vi "STP_22.1 - three_multiAO+dynamics.vi"() -> ()   [LabVIEW 2018]
uses:
  <vilib>/Math Plots/2D Math Plots/2D Compass/2D Compass XCtrl/2D Compass.xctl
  <vilib>/Utility/error.llb/DialogType.ctl
  <vilib>/Platform/TimedLoop/XDataNode/nitl_modes.ctl
  <vilib>/Platform/TimedLoop/XDataNode/timing_clust.ctl
  <vilib>/Platform/TimedLoop/XDataNode/wakeup.ctl
  <vilib>/DAQmx/write.llb/DAQmx Write (Analog 1D Wfm NChan NSamp).vi
  <vilib>/DAQmx/write.llb/DAQmx Write (Analog 2D DBL NChan NSamp).vi
  <vilib>/DAQmx/create/timing.llb/DAQmx Create Timing Source (Frequency).vi
  <vilib>/Instr/_visa.llb/VISA Configure Serial Port (Instr).vi
  <vilib>/Math Plots/2D Math Plots/2D Compass/2D Compass Datatype/Public/Plot Helper (Vector).vi
  <vilib>/DAQmx/create/channels.llb/DAQmx Create Channel (AO-Voltage-Basic).vi
  <vilib>/DAQmx/configure/timing.llb/DAQmx Timing (Sample Clock).vi
  <vilib>/DAQmx/miscellaneous.llb/DAQmx Fill In Error Info.vi
  <vilib>/measure/matone.llb/Extract Single Tone Information 1 Chan.vi
  <vilib>/Platform/TimedLoop/XDataNode/XDataNode.xnode
  <vilib>/measure/NI_MABase.lvlib
  <resource>/objmgr/daqmx.rc
  <vilib>/Platform/TimedLoop/XDataNode/XDNodeRunTimeDep.lvlib
  <vilib>/measure/NI_MAPro.lvlib
  <vilib>/Math Plots/2D Math Plots/2D Compass/2D Compass Datatype/2D Compass Datatype.lvclass
  <vilib>/Analysis/NI_AALBase.lvlib
  <vilib>/Analysis/NI_AALPro.lvlib
panel:
  out "rocof0":dbl[](array[numeric])
  out "rocof1":dbl[](array[numeric])
  out "ROCOF measured":dbl[](array[numeric])
  out "ROCOF reference":dbl[](array[numeric])
  out "Media":dbl
  in  "stop":bool
  out "Frequency reference":dbl[](array[numeric])
  out "Frequency measured":dbl[](array[numeric])
  out "Angle reference":dbl[](array[numeric])
  out "Angle measured":dbl[](array[numeric])
  out "Voltage reference":dbl[](array[numeric])
  out "Voltage measured":dbl[](array[numeric])
  out "freq1":dbl[](array[numeric])
  out "freq0":dbl[](array[numeric])
  out "magnitude1":dbl[](array[numeric])
  out "magnitude0":dbl[](array[numeric])
  in  "last amp":dbl
  out "phases0":dbl[](array[numeric])
  out "phases1":dbl[](array[numeric])
  out "initialized array":dbl[](array[numeric])
  out "Sine phase":dbl
  in  "Tab Control":T1(tab)
  out "Interf.\nAmplitude (%)":dbl
  out "Interf.\nFrequency (Hz)":dbl
  out "Amplitude (%)":dbl
  out "Harmonic order":i32
  out "reset\nphase?":bool
  out "Samples":dbl
  out "Frequency (Hz)":dbl
  out "Phase (deg)":dbl format="%.4f"
  out "Amplitude (V)":dbl format="%.4g"
  in  "Tab Control 3":T2(tab)
  in  "Interference":bool
  in  "Interf. Frequency":dbl caption="Frequency"
  in  "Interf. Amplitude":dbl caption="Amplitude (%)"
  in  "Amplitude (%)":dbl=10.0
  in  "Order":i32=2
  in  "Harmonics":bool
  in  "phase 2":dbl
  in  "duty cycle (%)":dbl=1.0
  in  "Pulse frequency":dbl=25.0
  in  "Noise":bool
  in  "Amplitude (rms)":dbl=0.0035355 format="%0.6f"
  in  "reset signal":bool
  in  "Phase":dbl format="%#.4f"
  in  "Frequency":dbl=50.0 format="%#.4f"
  in  "Offset":dbl=1.5 format="%#.4f"
  in  "Amplitude":dbl=1.25 format="%#.4f"
  in  "Steps":dbl=50.0
  in  "Save without\nvariation":bool
  in  "Amp. (%) 4":dbl=10.0 caption="Amplitude (%)"
  in  "Frequency\ninterval 2":dbl=0.5 caption="Frequency\ninterval"
  in  "Final freq. 2":dbl=100.0 caption="Final freq."
  in  "Initial freq. 2":dbl=27.5 caption="Initial freq."
  in  "Interference\nauto variation":bool
  in  "Amp. (%) 3":dbl=10.0 caption="Amplitude (%)"
  in  "Order\ninterval":i32=1
  in  "Final order":i32=50
  in  "Initial order":i32=2
  in  "Harmonics\nauto variation":bool
  in  "Frequency\ninterval":dbl=0.1 format="%.4f"
  in  "Final freq.":dbl=55.0 format="%.4f"
  in  "Initial freq.":dbl=45.0 format="%.4f"
  in  "Freq. auto\nvariation":bool
  in  "Phase\ninterval":dbl=10.0 format="%.4f"
  in  "Final phase":dbl=180.0 format="%.4f"
  in  "Initial phase":dbl=-180.0 format="%.4f"
  in  "Phase auto\nvariation":bool
  in  "Amplitude\ninterval":dbl=0.05 format="%.4f"
  in  "Initial ampl.":dbl=0.125 format="%.4f"
  in  "Final ampl.":dbl=1.25 format="%.4f"
  in  "Ampl. auto\nvariation":bool
  in  "Boolean 2":bool
  in  "Dynamic tests?":bool
  in  "Final fmod":dbl=5.0
  in  "fmod interval":dbl=0.2
  in  "Initial fmod":dbl
  in  "Modulation\nauto variation":bool
  in  "Select test type":T3(ring)
  in  "Freq. Ramp":bool
  in  "ka":dbl=0.1
  in  "kx":dbl=0.1
  out "fmod (Hz)":dbl
  in  "fmod":dbl
  in  "Signal generation":bool=TRUE
  in  "File name":path=path "teste.txt"
  in  "Data save":bool
  in  "Boolean":bool
  in  "step time (s)":i32=2
  out "step?":bool
  out "Cycle visualization":dbl[](graph)
  in  "Boolean 3":bool
  out "Phasors visualization":refnum<class "2D Plot Datatype.lvclass">[](xcontrol) caption="2D Compass"
  in  "Directory":path=path "D:/Resultados"
  in  "Sampling rate":dbl=200000.0
  in  "Porta":refnum<visa-resource-name>="COM3"
  in  "baud rate (kB)":u32=115200
  in  "data bits (8)":u16=8
  in  "timeout (ms)":u32=5000
  in  "parity (0:none)":enum16{"None", "Odd", "Even", "Mark", "Space"}(ring)
  in  "flow control (0:none)":u16(ring) items=["None", "XON/XOFF", "RTS/CTS", "XON/XOFF & RTS/CTS", "DTR/DSR", "XON/XOFF & DTR/DSR"]
  in  "stop bits (10: 1 bit)":u16(ring)=10 items=["1.0"=10, "1.5"=15, "2.0"=20]
  in  "Serial communication":bool=TRUE
  out "read buffer":string
  out "floating point data":sgl[](array[numeric])
  in  "Interference 2":bool caption="Interference"
  in  "amplitude":dbl=1.0 caption="Amp. (%)" format="%#.4p"
  in  "Interf. Frequency 2":dbl=10.0 caption="Frequency (Hz)"
  in  "Harmonics 2":bool caption="Harmonics"
  in  "Amp. (%) 2":dbl=10.0 caption="Amp. (%)"
  in  "Order 2":i32=3 caption="Order"
  out "Frequency":dbl
  in  "Offset 2":dbl=1.5 caption="Offset"
  out "Phase (degrees) 2":dbl caption="Phase (°)" format="%.4f"
  in  "Amplitude 2":dbl=1.25 caption="Amplitude"
  in  "Frequency 2":dbl=50.0 caption="Frequency"
  in  "Phase 2":dbl caption="Phase"
  in  "reset signal 2":bool caption="reset\nsignal"
  in  "Frequency\noff-set":dbl
  in  "Magnitude\noff-set":dbl
  in  "Magnitude\ncoefficient":dbl=1.0
  in  "Angle\noff-set":dbl
  out "mean rocof":dbl caption="ROCOF (Hz/s)" format="%.8g"
  out "max rocof":dbl caption="ROCOF (Hz/s)" format="%.8g"
  out "mean freq":dbl caption="Frequency (Hz)" format="%.8g"
  out "mean tve":dbl caption="TVE (%)" format="%.8g"
  out "mean phase":dbl caption="Phase (º)" format="%.8g"
  out "mean dev":dbl caption="Magnitude (%)" format="%.8g"
  out "max magnitude":dbl caption="Magnitude (%)" format="%.8g"
  out "max tve":dbl caption="TVE (%)" format="%.8g"
  out "max freq":dbl caption="Frequency (Hz)" format="%.8g"
  out "max phase":dbl caption="Phase (º)" format="%.8g"
  in  "Tab Control 2":T4(tab)
  out "Magnitude measures (V)":dbl[][](graph)
  in  "?":bool
  in  "RMS?":bool=TRUE
  out "Phase measures (º)":dbl[][](graph)
  in  "?":bool
  in  "Fase ref":enum16{"R", "S", "T"}(ring)
  out "Frequency measures (Hz)":dbl[][](graph)
  in  "?":bool
  out "ROCOF (Hz/s)":dbl[][](graph)
  in  "?":bool
  in  "?":bool
  out "Phase measures (º) 2":dbl[](graph)
  out "Iteration Duration 2":i64
  out "Finished Late? [i-1]":bool
  out "Iteration Duration":i64
  out "Iteration Duration 3":i64
  # "Synchrophasors Test Platform"
  # "A real-time platform for PMU development."
  # "Actual generation"
  # "PPS parameters"
  # "Noise"
  # "Sinusoid parameters"
  # "1 Hz/s"
  # "IEEE 754 conversion"
  # "Max errors:"
  # "Mean errors:"
  # "Signal generation parameters:"
  # "On-line corrections (received data):"
  # "This is a project developed by Flavio Lori Grando, during Masters in Electrical Engineering Graduate Program (PPGEE) of Federal University of Technology - Paraná, Brazil.\n\nContact: flavio.grando.eng@gmail.com"
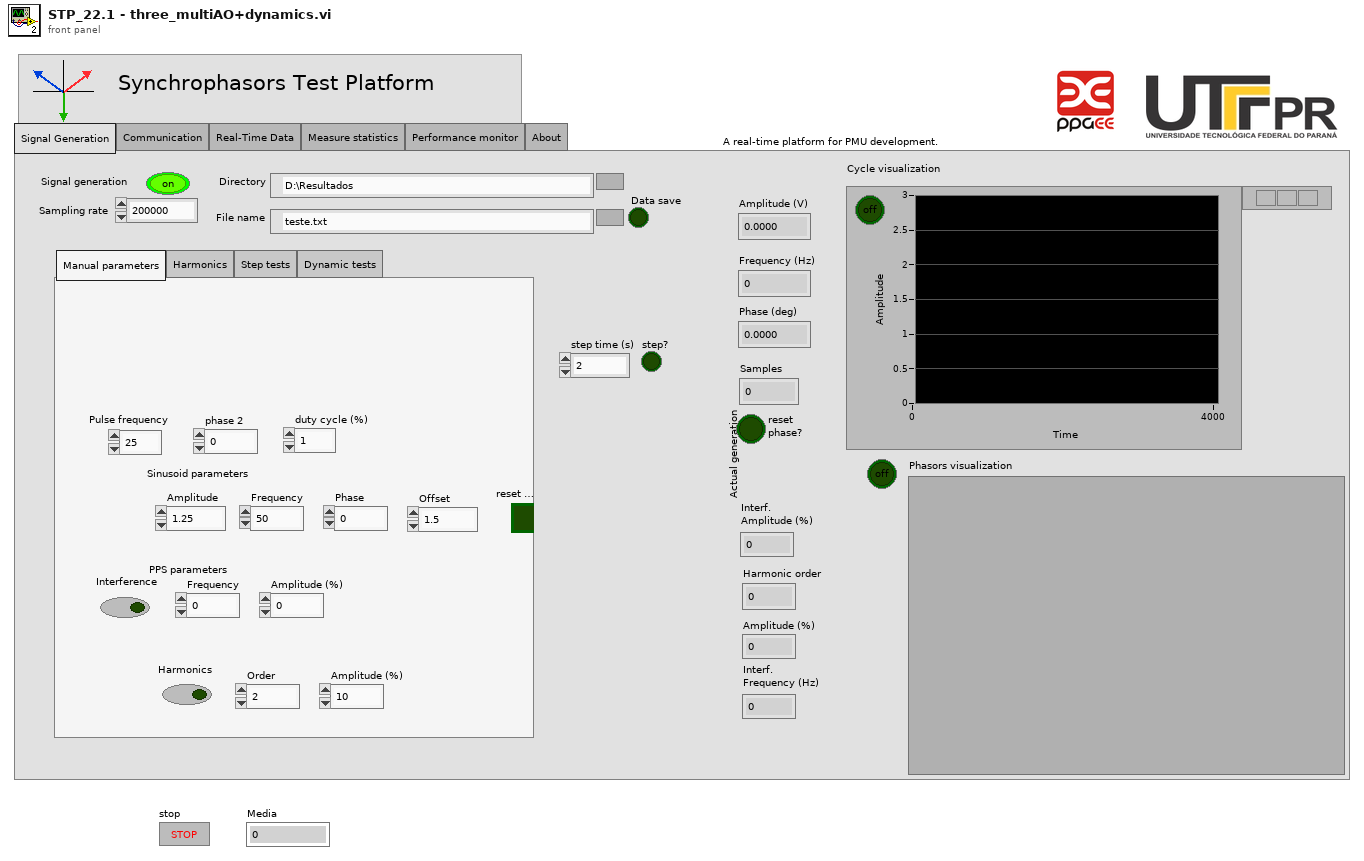
[diagram p1: front panel]
types:
  T1 = enum32{"Signal Generation", "Communication", "Real-Time Data", "Measure statistics", "Performance monitor", "About"}
  T2 = enum32{"Manual parameters", "Harmonics", "Step tests", "Dynamic tests"}
  T3 = enum16{"Amplitude modulation", "Phase modulation", "Frequency ramp"}
  T4 = enum32{"Magnitude", "Phase", "Frequency", "ROCOF", "Phase deviation"}
  T5 = enum16{"Sine Wave", "Triangle Wave", "Square Wave", "Sawtooth Wave"}
  T6 = typedef "XDNodeRunTimeDep.lvlib/nitl_modes.ctl" = enum32{"No Change", "Process missed periods, maintain original phase", "Discard missed periods, maintain original phase", "Process missed periods, ignore original phase", "Discard missed periods, ignore original phase"}
  T7 = cluster{"frequency":dbl, "amplitude":dbl, "phase":dbl}[]
  T8 = typedef "XDNodeRunTimeDep.lvlib/timing_clust.ctl" = cluster{"Expected End [f-1]":u64, "Actual End [f-1]":u64, "Finished Late? [f-1]":bool, "Expected End [i-1]":u64, "Actual End [i-1]":u64, "Finished Late? [i-1]":bool, "Expected Start [i]":u64, "Actual Start [i]":u64, "Expected Start [f]":u64, "Actual Start [f]":u64, "Source Name":string, "Structure Name":string, "Period":i64, "Deadline":i64, "Offset":i64, "Start":i64, "Priority":i32, "Timeout":i32, "Mode":T6, "Wakeup Reason":T9, "Error":errorcluster, "Source Type":string, "Secondary Source Type":string, "Global End Time":u64, "Global Start Time":u64, "Frame Duration":u64, "Iteration Duration":u64, "Assigned CPU":i32, "I/O Scan Engine Mode":u32}
  T9 = typedef "XDNodeRunTimeDep.lvlib/wakeup.ctl" = enum32{"Normal", "Aborted", "Asynchronous wakeup", "Timing source error", "Timed loop error", "Timeout"}
  T10 = typedef "DialogType.ctl" = u16
  T11 = cluster{"Sampling rate":dbl, "Sampling rate":dbl}
  T12 = enum16{"open", "replace", "create", "open or create", "replace or create", "replace or create with confirmation"}
  T13 = cluster{"max ref":dbl, "min ref":dbl, "mean ref":dbl, "max dev":dbl, "min dev":dbl, "mean dev":dbl, "max meas":dbl, "min meas":dbl, "mean meas":dbl}
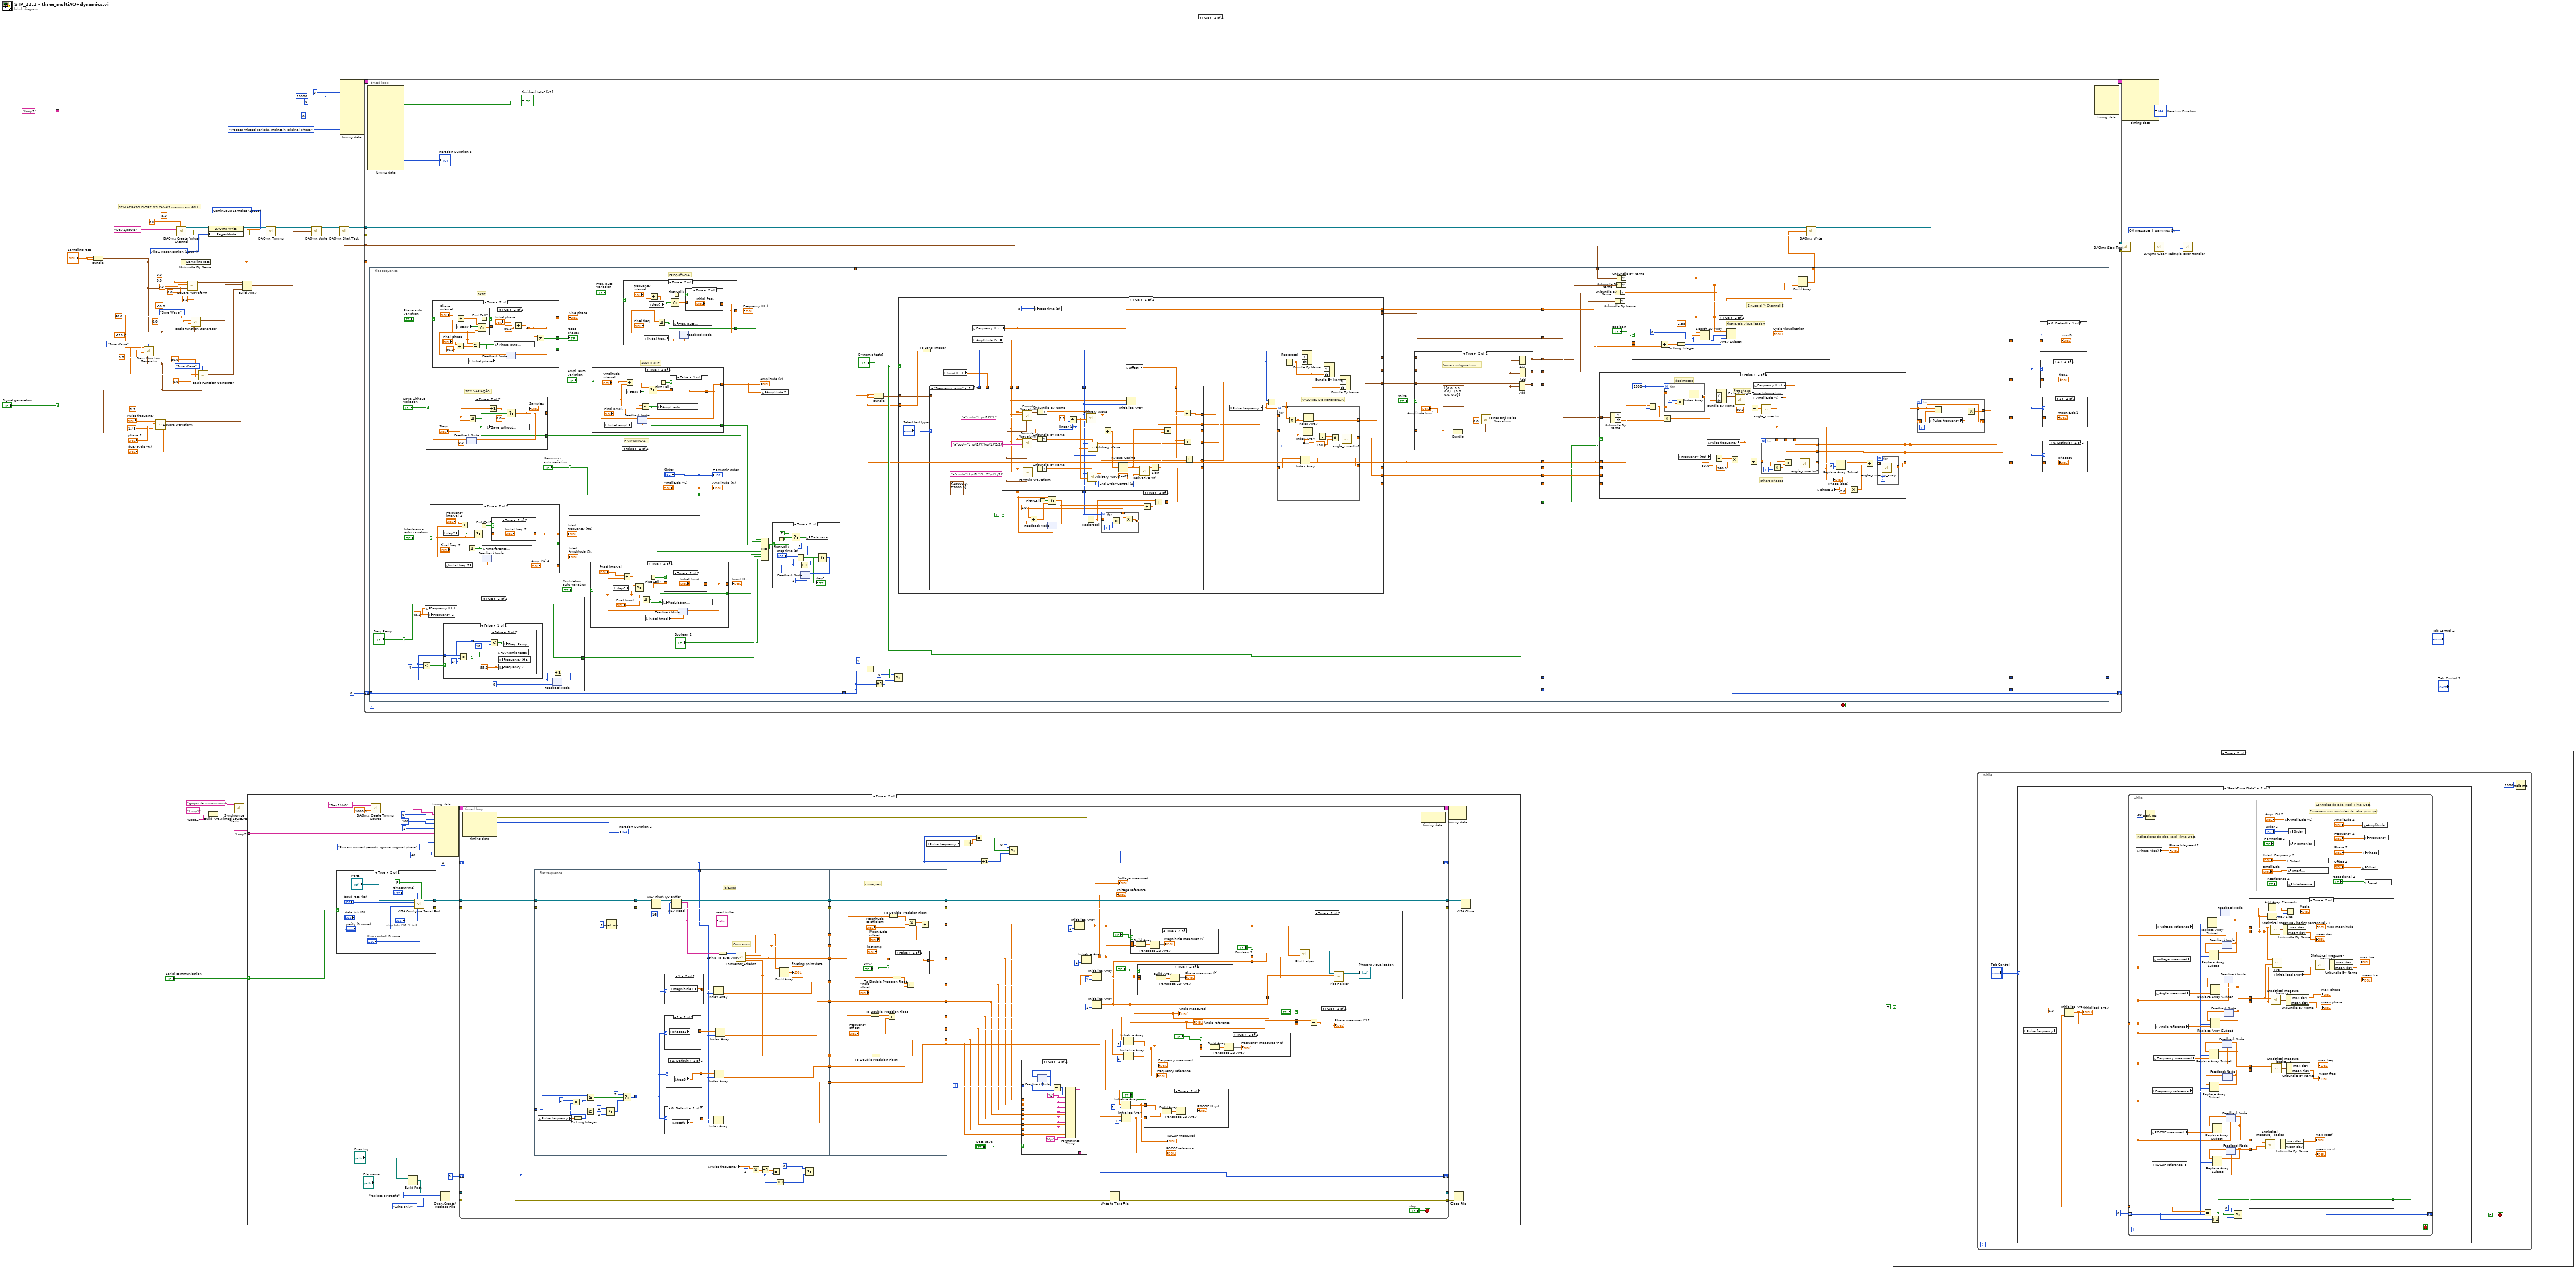
[diagram p0: block diagram]
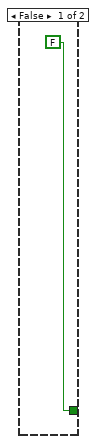
[diagram p4: hidden frame]
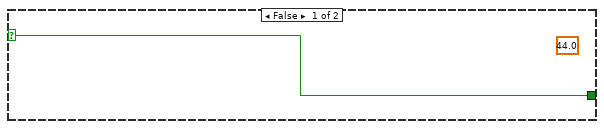
[diagram p7: hidden frame]
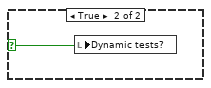
[diagram p8: hidden frame]
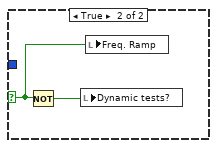
[diagram p9: hidden frame]
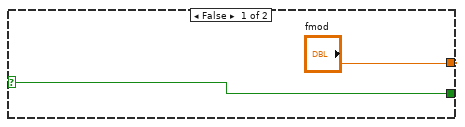
[diagram p10: hidden frame]
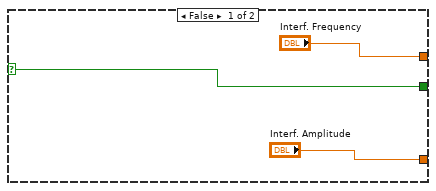
[diagram p12: hidden frame]
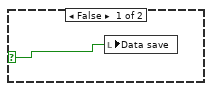
[diagram p14: hidden frame]
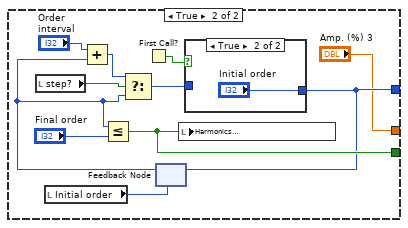
[diagram p15: hidden frame]
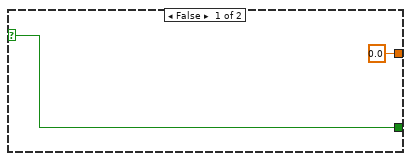
[diagram p17: hidden frame]
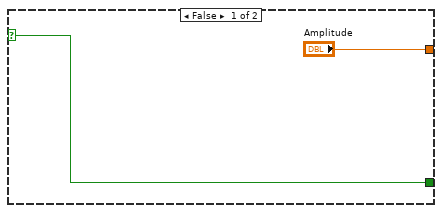
[diagram p18: hidden frame]
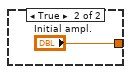
[diagram p19: hidden frame]
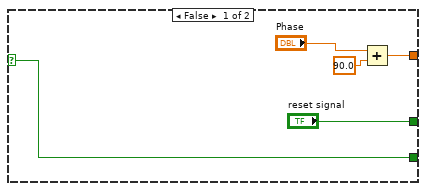
[diagram p20: hidden frame]
diagram:
  n1 = case shown="True" "Signal generation" {
    tunnel: "Loop1" -> [_ w33]
    frame False {
    }
    frame True {
      w20 = 60.0 ("frequency")
      w61 = 10097 items=["Allow Regeneration"=10097, "Do Not Allow Regeneration"=10158] ("RegenMode")
      w64 = 10123 items=["Finite Samples"=10178, "Continuous Samples"=10123] ("sample mode")
      w65 = T10 3 items=["no dialog", "OK message", "continue or stop message", "OK message + warnings", "continue/stop + warnings"] ("type of dialog (OK msg:1)")
      # "SEM ATRASO ENTRE OS CANAIS mesmo em 60Hz"
      n2 = Bundle("Sampling rate"="Sampling rate", "Sampling rate"="Sampling rate") -> (w11:T11)  [unwired: 1 in]
      n3 = call <vilib>:"Basic Function Generator.vi"("sampling info"=w11, "signal type"=T5."Sine Wave" ("signal type 4"), "phase"=-210.0 ("offset 4"), "amplitude"=0.0 ("amplitude 3"), "frequency"=w20) -> ("signal out"=w25:waveform(dbl))  [unwired: 4 in, 2 out]
      n4 = call <vilib>:"Square Waveform.vi"("duty cycle (%)"="duty cycle (%)", "offset"=1.5, "sampling info"=w11, "phase"="phase 2", "amplitude"=1.45, "frequency"="Pulse frequency") -> ("signal out"=w29:waveform(dbl))  [unwired: 4 in, 1 out]
      n5 = call-poly <vilib>:"DAQmx Create Virtual Channel.vi"("maximum value"=8.0 ("Maximum Value"), "minimum value"=-8.0 ("Minimum Value"), "physical channels"=tag "Dev1/ao0:3" ("Physical Channel")) -> ("task out"=w40:refnum<k21>, "error out"=w41:errorcluster)  [unwired: 11 in]
      n6 = Unbundle By Name(w11) -> ("Sampling rate"=w10:dbl)
      n7 = call <vilib>:"Square Waveform.vi"("duty cycle (%)"=5.0, "offset"=0.0, "sampling info"=w11, "phase"=0.0, "amplitude"=0.0, "frequency"=0.0) -> ("signal out"=w31:waveform(dbl))  [unwired: 4 in, 1 out]
      n8 = call <vilib>:"Basic Function Generator.vi"("sampling info"=w11, "signal type"=T5."Sine Wave" ("signal type 4"), "phase"=-90.0 ("offset 4"), "amplitude"=0.0 ("amplitude 3"), "frequency"=w20) -> ("signal out"=w32:waveform(dbl))  [unwired: 4 in, 2 out]
      n9 = call <vilib>:"Basic Function Generator.vi"("sampling info"=w11, "signal type"=T5."Sine Wave" ("signal type 4"), "phase"=30.0 ("offset 4"), "amplitude"=0.0 ("amplitude 3"), "frequency"=w20) -> ("signal out"=w21:waveform(dbl))  [unwired: 4 in, 2 out]
      n10 = property class="DAQmx Write"(reference=w40, error in=w41, "RegenMode"=w61) -> (reference out=w14:refnum<k21>, error out=w62:errorcluster)
      n11 = Build Array(w31, w32, w25, w21) -> (w34:waveform(dbl)[])
      n12 = call-poly <vilib>:"DAQmx Timing.vi"("task/channels in"=w14, "sample mode"=w64, "rate"=w10, "error in"=w62) -> ("task out"=w36:refnum<k21>, "error out"=w35:errorcluster)  [unwired: 10 in]
      n13 = call-poly <vilib>:"DAQmx Write.vi"("task/channels in"=w36, "data"=w34, "error in"=w35) -> ("task out"=w45:refnum<k21>, "error out"=w46:errorcluster)  [unwired: 10 in, 1 out]
      n14 = call <vilib>:"DAQmx Start Task.vi"("task/channels in"=w45, "error in"=w46) -> ("task out"=w37:refnum<k21>, "error out"=w38:errorcluster)  [unwired: 12 in]
      n15 = node-c288(i64 0 ("Period"), 10000 ("Priority"), 0 ("Processor"), w33, i64 0 ("Deadline"), nitl_modes."Process missed periods, maintain original phase" ("Mode")) -> (w69:T8)  [unwired: 4 in]
      n16 = timed-loop {
        tunnel: w37 -> [w74]
        tunnel: [w91] -> w54
        tunnel: [w90] -> w53
        timing: w69 -> [_]
        timing-out: [_] -> w68
        shift-right: [w98] -> _
        shift-left: 0 -> [w78]
        tunnel: w38 -> [w92]
        tunnel: w29 -> [w73]
        tunnel: w10 -> [w70]
        stop <- _ stop-if-true
        n17 = node-c288() -> (→"Finished Late? [i-1]":bool, →"Iteration Duration 3":i64)  [unwired: 1 in, 15 out]
        n18 = flat-sequence {
          tunnel: w78 -> [w122]
          tunnel: [w122] -> w88
          tunnel: [w278] -> w89
          tunnel: w88 -> [w277]
          tunnel: [w277] -> w87
          tunnel: [w264] -> w86
          tunnel: [w283] -> w85
          tunnel: [w273] -> w83
          tunnel: [w272] -> w82
          tunnel: [w274] -> w81
          tunnel: [w276] -> w80
          tunnel: [w268] -> w77
          tunnel: [w266] -> w76
          tunnel: [w267] -> w75
          tunnel: ["Dynamic tests?"] -> w71
          tunnel: w70 -> [w264]
          tunnel: [w576] -> w97
          tunnel: [w574] -> w96
          tunnel: [w567] -> w95
          tunnel: [w555] -> w94
          tunnel: w89 -> [w576]
          tunnel: w87 -> [w575]
          tunnel: [w575] -> w93
          tunnel: [w571] -> w72
          tunnel: w86 -> [w573]
          tunnel: w85 -> [w572]
          tunnel: [w554] -> w84
          tunnel: w83 -> [w566]
          tunnel: w82 -> [w565]
          tunnel: w81 -> [w560]
          tunnel: w80 -> [w570]
          tunnel: w77 -> [w569]
          tunnel: w76 -> [w556]
          tunnel: w75 -> [w568]
          tunnel: w73 -> [w559]
          tunnel: w71 -> [w557]
          tunnel: w97 -> [w646]
          tunnel: [w646] -> w98
          tunnel: w96 -> [w645]
          tunnel: w95 -> [w644]
          tunnel: w94 -> [w643]
          tunnel: w93 -> [w642]
          tunnel: w84 -> [w641]
          frame #0 {
            # "HARMONICAS"
            # "SEM VARIA敲O"
            # "FASE"
            # "FREQUÊNCIA"
            # "AMPLITUDE"
            n19 = case shown="True" "Freq. Ramp" {
              selector: "Freq. Ramp" -> [w128 w130]
              tunnel: [w128 w130] -> w101
              frame False {
                (unwired) 44.0 ("Initial freq. 3")
              }
              frame True {
                w129 = 45.0 ("Frequency")
                n20 = local write "Frequency (Hz)"(w129) -> ()
                n21 = local write "Frequency 2"(w129) -> ()
                n22 = feedback #1(0) -> (w132:i32)
                n23 = Less?(x=w132, y=4) -> (x < y?=w131:bool)
                n24 = case shown="False" w131 {
                  selector: w131 -> [_ w145]
                  tunnel: w132 -> [w137 _]
                  frame False {
                    n25 = Less?(x=w137, y=14) -> (x < y?=w136:bool)
                    n26 = case shown="False" w136 {
                      selector: w136 -> [w139 w144]
                      tunnel: w137 -> [w142 _]
                      frame False {
                        w140 = 55.0 ("Frequency")
                        n27 = Less?(x=w142, y=18) -> (x < y?=w141:bool)
                        n28 = local write "Dynamic tests?"(w139) -> ()
                        n29 = local write "Frequency (Hz)"(w140) -> ()
                        n30 = local write "Frequency 2"(w140) -> ()
                        n31 = local write "Freq. Ramp"(w141) -> ()
                      }
                      frame True {
                        n32 = local write "Dynamic tests?"(w144) -> ()
                      }
                    }
                  }
                  frame True {
                    n33 = Not(x=w145) -> (.not. x?=w146:bool)
                    n34 = local write "Dynamic tests?"(w146) -> ()
                    n35 = local write "Freq. Ramp"(w145) -> ()
                  }
                }
                n36 = Increment(x=w132) -> (x+1=w134:i32)
                n37 = feedback-in #1(w134) -> ()
              }
            }
            n38 = case shown="True" "Save without\nvariation" {
              selector: "Save without\nvariation" -> [w205 _]
              tunnel: [0.0 ("f") w208] -> _
              tunnel: [w205 w207] -> w116
              frame False {
              }
              frame True {
                n39 = feedback #2(0.0 ("f")) -> (w210:dbl)
                n40 = Less Or Equal?(x=w210, y="Steps") -> (x <= y?=w207:bool)
                n41 = local write "Save without\nvariation"(w207) -> ()
                n42 = Increment(x=w210) -> (x+1=w212:dbl)
                n43 = Select(t=w212, s=w207, f=0.0) -> (s? t:f=w208:dbl)
                "Samples" <- w208
                n44 = feedback-in #2(w208) -> ()
              }
            }
            n45 = case shown="True" "Interference\nauto variation" {
              selector: "Interference\nauto variation" -> [w161 _]
              tunnel: ["Interf. Frequency" w170] -> w108
              tunnel: ["Interf. Amplitude" "Amp. (%) 4"] -> w107
              tunnel: [w161 w164] -> w106
              frame False {
              }
              frame True {
                n46 = local read "step?"() -> (w167:bool)
                n47 = local read "Initial freq. 2"() -> (w171:dbl)
                n48 = First Call?() -> (First Call?: T/F=w174:bool)
                n49 = feedback #3(w171) -> (w166:dbl)
                n50 = Add(x="Frequency\ninterval 2", y=w166) -> (x+y=w168:dbl)
                n51 = Less Or Equal?(x=w166, y="Final freq. 2") -> (x <= y?=w164:bool)
                n52 = Select(t=w168, s=w167, f=w166) -> (s? t:f=w173:dbl)
                n53 = local write "Interference\nauto variation"(w164) -> ()
                n54 = case shown="True" w174 {
                  tunnel: [w175 "Initial freq. 2"] -> w170
                  tunnel: w173 -> [w175 _]
                  frame False {
                  }
                  frame True {
                  }
                }
                n55 = feedback-in #3(w170) -> ()
              }
            }
            "Interf.\nFrequency (Hz)" <- w108
            "Interf.\nAmplitude (%)" <- w107
            n56 = case shown="True" "Phase auto\nvariation" {
              selector: "Phase auto\nvariation" -> [w228 _]
              tunnel: ["reset signal" w243] -> w127
              tunnel: [w230 w242] -> w117
              tunnel: [w228 w237] -> w114
              frame False {
                n57 = Add(x="Phase", y=90.0) -> (x+y=w230:dbl)
              }
              frame True {
                n58 = Add(x="Final phase", y=90.0) -> (x+y=w239:dbl)
                n59 = local read "step?"() -> (w233:bool)
                n60 = local read "Initial phase"() -> (w241:dbl)
                n61 = First Call?() -> (First Call?: T/F=w244:bool)
                n62 = feedback #4(w241) -> (w235:dbl)
                n63 = Add(x="Phase\ninterval", y=w235) -> (x+y=w234:dbl)
                n64 = Less Or Equal?(x=w235, y=w239) -> (x <= y?=w237:bool)
                n65 = Select(t=w234, s=w233, f=w235) -> (s? t:f=w236:dbl)
                n66 = case shown="True" w244 {
                  tunnel: [w246 w247] -> w242
                  tunnel: w236 -> [w246 _]
                  frame False {
                  }
                  frame True {
                    n67 = Add(x="Initial phase", y=90.0) -> (x+y=w247:dbl)
                  }
                }
                n68 = local write "Phase auto\nvariation"(w237) -> ()
                n69 = feedback-in #4(w242) -> ()
                n70 = Not Equal?(x=w242, y=w235) -> (x != y?=w243:bool)
              }
            }
            "Sine phase" <- w117
            "reset\nphase?" <- w127
            n71 = case shown="False" "Harmonics\nauto variation" {
              selector: "Harmonics\nauto variation" -> [w190 _]
              tunnel: ["Order" w196] -> w112
              tunnel: [w190 w197] -> w110
              tunnel: ["Amplitude (%)" "Amp. (%) 3"] -> w111
              frame False {
              }
              frame True {
                n72 = local read "step?"() -> (w199:bool)
                n73 = local read "Initial order"() -> (w201:i32)
                n74 = First Call?() -> (First Call?: T/F=w198:bool)
                n75 = feedback #5(w201) -> (w194:i32)
                n76 = Add(x="Order\ninterval", y=w194) -> (x+y=w193:i32)
                n77 = Less Or Equal?(x=w194, y="Final order") -> (x <= y?=w197:bool)
                n78 = Select(t=w193, s=w199, f=w194) -> (s? t:f=w202:i32)
                n79 = local write "Harmonics\nauto variation"(w197) -> ()
                n80 = case shown="True" w198 {
                  tunnel: [w203 "Initial order"] -> w196
                  tunnel: w202 -> [w203 _]
                  frame False {
                  }
                  frame True {
                  }
                }
                n81 = feedback-in #5(w196) -> ()
              }
            }
            "Harmonic order" <- w112
            "Amplitude (%)" <- w111
            n82 = case shown="True" "Modulation\nauto variation" {
              selector: "Modulation\nauto variation" -> [w148 _]
              tunnel: [w148 w151] -> w104
              tunnel: ["fmod" w150] -> w103
              frame False {
              }
              frame True {
                n83 = local read "step?"() -> (w157:bool)
                n84 = local read "Initial fmod"() -> (w149:dbl)
                n85 = First Call?() -> (First Call?: T/F=w158:bool)
                n86 = feedback #6(w149) -> (w154:dbl)
                n87 = Add(x="fmod interval", y=w154) -> (x+y=w156:dbl)
                n88 = Select(t=w156, s=w157, f=w154) -> (s? t:f=w152:dbl)
                n89 = Less Or Equal?(x=w154, y="Final fmod") -> (x <= y?=w151:bool)
                n90 = local write "Modulation\nauto variation"(w151) -> ()
                n91 = case shown="True" w158 {
                  tunnel: [w159 "Initial fmod"] -> w150
                  tunnel: w152 -> [w159 _]
                  frame False {
                  }
                  frame True {
                  }
                }
                n92 = feedback-in #6(w150) -> ()
              }
            }
            "fmod (Hz)" <- w103
            n93 = case shown="True" "Ampl. auto\nvariation" {
              selector: "Ampl. auto\nvariation" -> [w214 _]
              tunnel: ["Amplitude" w223] -> w121
              tunnel: [w214 w218] -> w115
              frame False {
              }
              frame True {
                n94 = local read "Initial ampl."() -> (w222:dbl)
                n95 = local read "step?"() -> (w219:bool)
                n96 = feedback #7(w222) -> (w217:dbl)
                n97 = Add(x="Amplitude\ninterval", y=w217) -> (x+y=w221:dbl)
                n98 = Less Or Equal?(x=w217, y="Final ampl.") -> (x <= y?=w218:bool)
                n99 = Select(t=w221, s=w219, f=w217) -> (s? t:f=w220:dbl)
                n100 = local write "Ampl. auto\nvariation"(w218) -> ()
                n101 = First Call?() -> (First Call?: T/F=w224:bool)
                n102 = case shown="False" w224 {
                  tunnel: [w226 "Initial ampl."] -> w223
                  tunnel: w220 -> [w226 _]
                  frame False {
                  }
                  frame True {
                  }
                }
                n103 = feedback-in #7(w223) -> ()
              }
            }
            "Amplitude (V)" <- w121
            n104 = case shown="True" "Freq. auto\nvariation" {
              selector: "Freq. auto\nvariation" -> [w251 _]
              tunnel: ["Frequency" w258] -> w119
              tunnel: [w251 w256] -> w113
              frame False {
              }
              frame True {
                n105 = local read "Initial freq."() -> (w257:dbl)
                n106 = local read "step?"() -> (w252:bool)
                n107 = First Call?() -> (First Call?: T/F=w260:bool)
                n108 = feedback #8(w257) -> (w253:dbl)
                n109 = Add(x="Frequency\ninterval", y=w253) -> (x+y=w254:dbl)
                n110 = Less Or Equal?(x=w253, y="Final freq.") -> (x <= y?=w256:bool)
                n111 = Select(t=w254, s=w252, f=w253) -> (s? t:f=w255:dbl)
                n112 = local write "Freq. auto\nvariation"(w256) -> ()
                n113 = case shown="True" w260 {
                  tunnel: [w262 "Initial freq."] -> w258
                  tunnel: w255 -> [w262 _]
                  frame False {
                  }
                  frame True {
                  }
                }
                n114 = feedback-in #8(w258) -> ()
              }
            }
            "Frequency (Hz)" <- w119
            n115 = local write "Amplitude 2"(w121) -> ()
            n116 = Compound Arithmetic op=OR(w113, w114, w115, w116, w110, w106, w104, w101, "Boolean 2") -> (w118:bool)
            n117 = case shown="True" w118 {
              selector: w118 -> [w177 w186]
              frame False {
                n118 = local write "Data save"(w177) -> ()
              }
              frame True {
                n119 = First Call?() -> (First Call?: T/F=w188:bool)
                n120 = Select(t=TRUE, s=w188, f=w186) -> (s? t:f=w185:bool)
                n121 = feedback #9(1 ("f")) -> (w178:i32)
                n122 = Equal?(x="step time (s)", y=w178) -> (x = y?=w181:bool)
                "step?" <- w181
                n123 = Increment(x=w178) -> (x+1=w179:i32)
                n124 = local write "Data save"(w185) -> ()
                n125 = Select(t=1 ("f"), s=w181, f=w179) -> (s? t:f=w184:i32)
                n126 = feedback-in #9(w184) -> ()
              }
            }
          }
          frame #1 {
            n127 = Equal?(x=1, y=w277) -> (x = y?=w282:bool)
            n128 = Bundle("Sampling rate"=w264, "Sampling rate"=w264) -> (w284:T11)  [unwired: 1 in]
            n129 = Increment(x=w277) -> (x+1=w280:i32)
            n130 = Select(t=0, s=w282, f=w280) -> (s? t:f=w278:i32)
            n131 = case shown="True" "Dynamic tests?" {
              tunnel: w284 -> [w309 w498]
              tunnel: [w313 w500] -> w283
              tunnel: [w318 w492] -> w275
              tunnel: [w317 w491] -> w271
              tunnel: [w323 w487] -> w269
              tunnel: [_ w482] -> w276
              tunnel: w264 -> [w321 _]
              tunnel: [w312 _] -> w268
              tunnel: [w311 _] -> w267
              tunnel: [w302 _] -> w266
              frame True {
                # "VALORES DE REFERENCIA"
                n132 = To Long Integer(number=w321) -> (32bit integer=w315:i32)
                n133 = local read "fmod (Hz)"() -> (w310:dbl)
                n134 = local read "Frequency (Hz)"() -> (w313:dbl)
                n135 = local read "Amplitude (V)"() -> (w322:dbl)
                n136 = local write "step time (s)"(5) -> ()
                n137 = local read "Offset"() -> (w301:dbl)
                n138 = case shown="\"Frequency ramp\"" "Select test type" {
                  tunnel: w322 -> [w335 w380 w456]
                  tunnel: w313 -> [w332 w378 w442]
                  tunnel: w315 -> [_ w383 w435]
                  tunnel: [w349 w369 w451] -> w303
                  tunnel: [w329 w375 w433] -> w306
                  tunnel: [w327 w370 w444] -> w308
                  tunnel: [w326 w372 w443] -> w307
                  tunnel: w315 -> [w331 _ w431]
                  tunnel: [w343 w382 w441] -> w304
                  tunnel: w310 -> [w341 _ w436]
                  tunnel: w309 -> [w342 _ w434]
                  tunnel: [w334 w386 w433] -> w305
                  tunnel: w301 -> [w325 w374 _]
                  frame "Phase modulation" {
                    # "referencia"
                    n139 = call <vilib>:"Sine Waveform.vi"("sampling info"=w342, "phase"=-90.0, "amplitude"="ka", "frequency"=w341) -> ("signal out"=w345:waveform(dbl))  [unwired: 6 in, 1 out]
                    n140 = call <vilib>:"Sine Waveform.vi"("sampling info"=w342, "phase"=-180.0, "amplitude"="ka", "frequency"=w341) -> ("signal out"=w339:waveform(dbl))  [unwired: 6 in, 1 out]
                    n141 = Unbundle By Name(w345) -> ("Y"=w336:dbl[])
                    n142 = Unbundle By Name(w339) -> ("Y"=w338:dbl[])
                    n143 = Reciprocal(x=w331) -> (1/x=w333:dbl)
                    n144 = Multiply(x=w332, y=6.283185307179586) -> (x*y=w347:dbl)
                    n145 = Divide(x=6.283185307179586, y=3.0) -> (x/y=w352:dbl)
                    n146 = Multiply(x=w347, y=w333) -> (x*y=w348:dbl)
                    n147 = for {
                      N: w331 -> [_]
                      tunnel: w348 -> [w360]
                      tunnel: [w368] -> w355 mode=indexing
                      tunnel: [w357] -> w349 mode=indexing
                      tunnel: w352 -> [w365]
                      tunnel: [w364] -> w351 mode=indexing
                      tunnel: [w363] -> w350 mode=indexing
                      tunnel: w336 -> [w357] mode=indexing
                      tunnel: [w358] -> w334 mode=indexing
                      tunnel: w335 -> [w358]
                      i -> [w359]
                      n148 = Multiply(x=w360, y=w359) -> (x*y=w362:dbl)
                      n149 = Add(x=w362, y=w357) -> (x+y=w361:dbl)
                      n150 = Add(x=w361, y=w365) -> (x+y=w366:dbl)
                      n151 = Subtract(x=w361, y=w365) -> (x-y=w367:dbl)
                      n152 = Cosine(x=w366) -> (cos(x)=w364:dbl)
                      n153 = Cosine(x=w367) -> (cos(x)=w363:dbl)
                      n154 = Cosine(x=w361) -> (cos(x)=w368:dbl)
                    }
                    n155 = Multiply(x=w338, y=w341) -> (x*y=w344:dbl[])
                    n156 = Multiply(x=w335, y=w350) -> (x*y=w328:dbl[])
                    n157 = Multiply(x=w335, y=w351) -> (x*y=w324:dbl[])
                    n158 = Multiply(x=w335, y=w355) -> (x*y=w330:dbl[])
                    n159 = Subtract(x=w332, y=w344) -> (x-y=w343:dbl[])
                    n160 = Add(x=w325, y=w330) -> (x+y=w329:dbl[])
                    n161 = Add(x=w325, y=w324) -> (x+y=w326:dbl[])
                    n162 = Add(x=w325, y=w328) -> (x+y=w327:dbl[])
                  }
                  frame "Frequency ramp" {
                    w389 = u16 0 items=["2nd Order Central", "4th Order Central", "Forward", "Backward"] ("method")
                    w384 = 1 items=["none", "linear"] ("interpolation")
                    w395 = cluster{"Fs":dbl, "#s":dbl} {"Fs"=25000.0, "#s"=25000.0} ("sampling info")
                    n163 = case shown="True" TRUE {
                      tunnel: w383 -> [w405 w423]
                      tunnel: [w402 w420] -> w382
                      tunnel: w378 -> [w406 w418]
                      frame False {
                        n164 = First Call?() -> (First Call?: T/F=w408:bool)
                        n165 = feedback #10(w406) -> (w409:dbl)
                        n166 = Decrement(x=w409) -> (x-1=w407:dbl)
                        n167 = Select(t=w406, s=w408, f=w407) -> (s? t:f=w410:dbl)
                        n168 = feedback-in #10(w410) -> ()
                        n169 = Reciprocal(x=w405) -> (1/x=w403:dbl)
                        n170 = for {
                          N: w405 -> [_]
                          tunnel: w403 -> [w414]
                          tunnel: [w413] -> w411 mode=indexing
                          i -> [w412]
                          n171 = Multiply(x=w414, y=w412) -> (x*y=w413:dbl)
                        }
                        n172 = Subtract(x=w410, y=w411) -> (x-y=w404:dbl[])
                        n173 = Subtract(x=w404, y=w403) -> (x-y=w402:dbl[])
                      }
                      frame True {
                        w415 = 1.0 ("x")
                        n174 = First Call?() -> (First Call?: T/F=w425:bool)
                        n175 = feedback #11(w418) -> (w417:dbl)
                        n176 = Add(x=w415, y=w417) -> (x+y=w416:dbl)
                        n177 = Select(t=w418, s=w425, f=w416) -> (s? t:f=w424:dbl)
                        n178 = feedback-in #11(w424) -> ()
                        n179 = Reciprocal(x=w423) -> (1/x=w419:dbl)
                        n180 = for {
                          N: w423 -> [_]
                          tunnel: w419 -> [w430]
                          tunnel: [w427] -> w422 mode=indexing
                          tunnel: w415 -> [w426]
                          i -> [w429]
                          n181 = Multiply(x=w430, y=w429) -> (x*y=w428:dbl)
                          n182 = Multiply(x=w426, y=w428) -> (x*y=w427:dbl)
                        }
                        n183 = Add(x=w424, y=w422) -> (x+y=w421:dbl[])
                        n184 = Add(x=w419, y=w421) -> (x+y=w420:dbl[])
                      }
                    }
                    n185 = call <vilib>:"Formula Waveform.vi"("sampling info"=w395, "formula"="a*cos(w*t+pi(1)*t*t)", "amplitude"=w380, "frequency"=w378) -> ("signal out"=w400:waveform(dbl))  [unwired: 6 in, 1 out]
                    n186 = call <vilib>:"Formula Waveform.vi"("sampling info"=w395, "formula"="a*cos(w*t+pi(1)*t*t-pi(1)*2/3)", "amplitude"=w380, "frequency"=w378) -> ("signal out"=w397:waveform(dbl))  [unwired: 6 in, 1 out]
                    n187 = call <vilib>:"Formula Waveform.vi"("sampling info"=w395, "formula"="a*cos(w*t+pi(1)*t*t+2*pi(1)/3)", "amplitude"=w380, "frequency"=w378) -> ("signal out"=w396:waveform(dbl))  [unwired: 6 in, 1 out]
                    n188 = Unbundle By Name(w397) -> ("Y"=w392:dbl[])
                    n189 = Unbundle By Name(w396) -> ("Y"=w391:dbl[])
                    n190 = Unbundle By Name(w400) -> ("Y"=w393:dbl[])
                    n191 = Divide(x=1.0, y=w383) -> (x/y=w390:dbl)
                    n192 = call <vilib>:"Arbitrary Wave.vi"("interpolation"=w384, "Wave Table"=w393, "frequency"=w390, "samples"=w383) -> ("arbitrary wave"=w376:dbl[])  [unwired: 3 in, 2 out]
                    n193 = call <vilib>:"Arbitrary Wave.vi"("interpolation"=w384, "Wave Table"=w391, "frequency"=w390, "samples"=w383) -> ("arbitrary wave"=w373:dbl[])  [unwired: 3 in, 2 out]
                    n194 = call <vilib>:"Arbitrary Wave.vi"("interpolation"=w384, "Wave Table"=w392, "frequency"=w390, "samples"=w383) -> ("arbitrary wave"=w371:dbl[])  [unwired: 3 in, 2 out]
                    n195 = Divide(x=w376, y=w380) -> (x/y=w379:dbl[])
                    n196 = Inverse Cosine(1:w379) -> (0:w381:dbl[])
                    n197 = Initialize Array(w380, w383) -> (w386:dbl[])
                    n198 = call <vilib>:"Derivative x(t).vi"("method"=w389, "dt"=1e-05, "X"=w381) -> ("dX/dt"=w387:dbl[])  [unwired: 7 in, 1 out]
                    n199 = Sign(1:w387) -> (0:w385:dbl[])
                    n200 = Multiply(x=w381, y=w385) -> (x*y=w369:dbl[])
                    n201 = Add(x=w374, y=w376) -> (x+y=w375:dbl[])
                    n202 = Add(x=w374, y=w371) -> (x+y=w370:dbl[])
                    n203 = Add(x=w374, y=w373) -> (x+y=w372:dbl[])
                  }
                  frame "Amplitude modulation" {
                    n204 = call <vilib>:"Sine Waveform.vi"("sampling info"=w434, "phase"=90.0 ("phase in"), "amplitude"="kx", "frequency"=w436) -> ("signal out"=w438:waveform(dbl))  [unwired: 6 in, 1 out]
                    n205 = Unbundle By Name(w438) -> ("Y"=w437:dbl[])
                    n206 = Add(x=w456, y=w437) -> (x+y=w445:dbl[])
                    n207 = Reciprocal(x=w431) -> (1/x=w432:dbl)
                    n208 = Multiply(x=w442, y=6.283185307179586) -> (x*y=w454:dbl)
                    n209 = Divide(x=6.283185307179586, y=3.0) -> (x/y=w448:dbl)
                    n210 = Multiply(x=w454, y=w432) -> (x*y=w453:dbl)
                    n211 = for {
                      N: w435 -> [_]
                      tunnel: w453 -> [w464]
                      tunnel: [w465] -> w452 mode=indexing
                      tunnel: [w461] -> w451 mode=indexing
                      tunnel: w448 -> [w460]
                      tunnel: [w459] -> w447 mode=indexing
                      tunnel: [w458] -> w446 mode=indexing
                      tunnel: [w457] -> w441 mode=indexing
                      tunnel: w442 -> [w457]
                      i -> [w466]
                      n212 = Multiply(x=w464, y=w466) -> (x*y=w461:dbl)
                      n213 = Add(x=w461, y=w460) -> (x+y=w462:dbl)
                      n214 = Subtract(x=w461, y=w460) -> (x-y=w463:dbl)
                      n215 = Cosine(x=w462) -> (cos(x)=w459:dbl)
                      n216 = Cosine(x=w463) -> (cos(x)=w458:dbl)
                      n217 = Cosine(x=w461) -> (cos(x)=w465:dbl)
                    }
                    n218 = Multiply(x=w445, y=w446) -> (x*y=w444:dbl[])
                    n219 = Multiply(x=w445, y=w447) -> (x*y=w443:dbl[])
                    n220 = Multiply(x=w445, y=w452) -> (x*y=w433:dbl[])
                  }
                }
                n221 = local read "Pulse frequency"() -> (w320:dbl)
                n222 = Divide(x=w315, y=w320) -> (x/y=w319:dbl)
                n223 = for {
                  N: w320 -> [_]
                  tunnel: w303 -> [w480]
                  tunnel: w319 -> [w478]
                  tunnel: [w471] -> w312 mode=indexing
                  tunnel: w305 -> [w472]
                  tunnel: [w470] -> w311 mode=indexing
                  tunnel: w304 -> [w469]
                  tunnel: [w467] -> w302 mode=indexing
                  i -> [w479]
                  n224 = Multiply(x=w478, y=w479) -> (x*y=w468:dbl)
                  n225 = Index Array(array=w469, index=w468) -> (element=w467:dbl)
                  n226 = Index Array(array=w480, index=w468) -> (element=w475:dbl)
                  n227 = Index Array(array=w472, index=w468) -> (element=w471:dbl)
                  n228 = Divide(x=w475, y=3.141592653589793) -> (x/y=w474:dbl)
                  n229 = Multiply(x=w474, y=180.0) -> (x*y=w473:dbl)
                  n230 = call "angle_corrector2.vi"("angle"=w473) -> ("angle corrected"=w470:dbl)  [unwired: 10 in]
                }
                n231 = Reciprocal(x=w315) -> (1/x=w316:dbl)
                n232 = Bundle By Name("Y"=w306, "dt"=w316) -> (w323:waveform(dbl))  [unwired: 1 in]
                n233 = Bundle By Name("Y"=w308, "dt"=w316) -> (w318:waveform(dbl))  [unwired: 1 in]
                n234 = Bundle By Name("Y"=w307, "dt"=w316) -> (w317:waveform(dbl))  [unwired: 1 in]
              }
              frame False {
                # "Sinusoid configurations"
                n235 = local read "reset\nphase?"() -> (w499:bool)
                n236 = local read "Frequency (Hz)"() -> (w500:dbl)
                n237 = local read "Amplitude (V)"() -> (w501:dbl)
                n238 = local read "Sine phase"() -> (w505:dbl)
                n239 = local write "Offset 2"("Offset") -> ()
                n240 = Subtract(x=w505, y=120.0) -> (x-y=w507:dbl)
                n241 = call <vilib>:"Sine Waveform.vi"("offset"="Offset", "sampling info"=w498, "reset signal"=w499, "phase"=w505, "amplitude"=w501, "frequency"=w500) -> ("signal out"=w485:waveform(dbl))  [unwired: 4 in, 1 out]
                n242 = Subtract(x=w505, y=240.0) -> (x-y=w504:dbl)
                n243 = call <vilib>:"Sine Waveform.vi"("offset"="Offset", "sampling info"=w498, "reset signal"=w499, "phase"=w507, "amplitude"=w501, "frequency"=w500) -> ("signal out"=w484:waveform(dbl))  [unwired: 4 in, 1 out]
                n244 = call <vilib>:"Sine Waveform.vi"("offset"="Offset", "sampling info"=w498, "reset signal"=w499, "phase"=w504, "amplitude"=w501, "frequency"=w500) -> ("signal out"=w483:waveform(dbl))  [unwired: 4 in, 1 out]
                n245 = case shown="\"R\"" "Fase ref" {
                  tunnel: w485 -> [_ _ w512]
                  tunnel: w484 -> [w510 _ _]
                  tunnel: w483 -> [_ w511 _]
                  tunnel: [w510 w511 w512] -> w482
                  frame "S" {
                  }
                  frame "T" {
                  }
                  frame "R" {
                  }
                }
                n246 = local read "Harmonics\nauto variation"() -> (w494:bool)
                n247 = local read "Amplitude (V)"() -> (w493:dbl)
                n248 = Or(x=w494, y="Harmonics") -> (x .or. y?=w496:bool)
                n249 = case shown="True" w496 {
                  tunnel: w483 -> [w535 w548]
                  tunnel: [w535 w547] -> w509
                  tunnel: w498 -> [_ w546]
                  tunnel: w484 -> [w534 w544]
                  tunnel: w485 -> [w533 w543]
                  tunnel: [w534 w541] -> w503
                  tunnel: [w533 w540] -> w502
                  tunnel: [w532 w537] -> w497
                  tunnel: w493 -> [w532 w537]
                  frame False {
                  }
                  frame True {
                    n250 = local read "Amplitude (%)"() -> (w539:dbl)
                    n251 = local read "Harmonic order"() -> (w545:i32)
                    n252 = local read "Frequency (Hz)"() -> (w538:dbl)
                    n253 = Divide(x=w539, y=100.0) -> (x/y=w550:dbl)
                    n254 = Multiply(x=w538, y=w545) -> (x*y=w553:dbl)
                    "Frequency" <- w553
                    n255 = Multiply(x=w537, y=w550) -> (x*y=w549:dbl)
                    n256 = call <vilib>:"Sine Waveform.vi"("sampling info"=w546, "phase"=0.0, "amplitude"=w549, "frequency"=w553) -> ("error out"=w536:errorcluster, "signal out"=w542:waveform(dbl))  [unwired: 6 in]
                    n257 = Add(1:w542, 2:w543, 4:w536) -> (0:w540:waveform(dbl))  [unwired: 1 out]
                    n258 = Add(1:w542, 2:w544, 4:w536) -> (0:w541:waveform(dbl))  [unwired: 1 out]
                    n259 = Add(1:w542, 2:w548, 4:w536) -> (0:w547:waveform(dbl))  [unwired: 1 out]
                  }
                }
                n260 = local read "Interference\nauto variation"() -> (w488:bool)
                n261 = Or(x="Interference", y=w488) -> (x .or. y?=w490:bool)
                n262 = case shown="True" w490 {
                  tunnel: w497 -> [_ w528]
                  tunnel: w498 -> [_ w527]
                  tunnel: w509 -> [w515 w526]
                  tunnel: [w515 w525] -> w491
                  tunnel: w503 -> [w514 w524]
                  tunnel: w502 -> [w513 w522]
                  tunnel: [w514 w523] -> w492
                  tunnel: [w513 w520] -> w487
                  frame False {
                  }
                  frame True {
                    n263 = local read "Interf.\nFrequency (Hz)"() -> (w518:dbl)
                    n264 = local read "Interf.\nAmplitude (%)"() -> (w519:dbl)
                    n265 = Divide(x=w519, y=100.0) -> (x/y=w530:dbl)
                    n266 = Multiply(x=w528, y=w530) -> (x*y=w529:dbl)
                    n267 = call <vilib>:"Sine Waveform.vi"("sampling info"=w527, "phase"=0.0, "amplitude"=w529, "frequency"=w518) -> ("error out"=w516:errorcluster, "signal out"=w521:waveform(dbl))  [unwired: 6 in]
                    n268 = Add(1:w521, 2:w524, 4:w516) -> (0:w523:waveform(dbl))  [unwired: 1 out]
                    n269 = Add(1:w521, 2:w522, 4:w516) -> (0:w520:waveform(dbl))  [unwired: 1 out]
                    n270 = Add(1:w521, 2:w526, 4:w516) -> (0:w525:waveform(dbl))  [unwired: 1 out]
                  }
                }
              }
            }
            n271 = case shown="True" "Noise" {
              tunnel: w275 -> [w286 w299]
              tunnel: w269 -> [w287 w298]
              tunnel: [w287 w297] -> w274
              tunnel: [w286 w296] -> w273
              tunnel: [w285 w295] -> w272
              tunnel: w271 -> [w285 w294]
              tunnel: w264 -> [_ w290]
              frame False {
              }
              frame True {
                # "Noise configurations"
                n272 = Bundle("Sampling rate"=w290, "Sampling rate"=w290) -> (w293:T11)  [unwired: 1 in]
                n273 = call <vilib>:"Tones and Noise Waveform.vi"("sampling info"=w293, "offset"=0.0, "noise (rms)"="Amplitude (rms)", "tones"=T7 [{"frequency"=0.0, "amplitude"=0.0, "phase"=0.0}, {"frequency"=0.0, "amplitude"=0.0, "phase"=0.0}]) -> ("signal out"=w288:waveform(dbl))  [unwired: 6 in, 1 out]
                n274 = Add(1:w288, 2:w294) -> (0:w295:waveform(dbl))  [unwired: 1 in, 1 out]
                n275 = Add(1:w288, 2:w298) -> (0:w297:waveform(dbl))  [unwired: 1 in, 1 out]
                n276 = Add(1:w288, 2:w299) -> (0:w296:waveform(dbl))  [unwired: 1 in, 1 out]
              }
            }
          }
          frame #2 {
            # "Sinusoid > Channel 3"
            n277 = case shown="False" w557 {
              tunnel: [w593 w607] -> w567
              tunnel: [w592 w594] -> w574
              tunnel: w573 -> [_ w606]
              tunnel: [w591 w605] -> w555
              tunnel: w570 -> [_ w600]
              tunnel: w569 -> [w593 _]
              tunnel: w556 -> [w591 _]
              tunnel: w568 -> [w592 _]
              frame True {
              }
              frame False {
                w622 = 1000
                # "others phases"
                # "first phase"
                # "decimacao"
                n278 = Unbundle By Name(w600) -> ("Y"=w601:dbl[], "dt"=w602:dbl)
                n279 = Divide(x=w606, y=w622) -> (x/y=w621:dbl)
                n280 = Multiply(x=w621, y=w602) -> (x*y=w624:dbl)
                n281 = for {
                  N: w622 -> [_]
                  tunnel: w601 -> [w640]
                  tunnel: [w637] -> w625 mode=indexing
                  tunnel: w621 -> [w636]
                  i -> [w638]
                  n282 = Multiply(x=w638, y=w636) -> (x*y=w639:dbl)
                  n283 = Index Array(array=w640, index=w639) -> (element=w637:dbl)
                }
                n284 = local read "Frequency (Hz)"() -> (w615:dbl)
                n285 = local read "Pulse frequency"() -> (w611:dbl)
                n286 = Subtract(x=w615, y=50.0) -> (x-y=w614:dbl)
                n287 = Bundle By Name("Y"=w625, "dt"=w624) -> (w623:waveform(dbl))  [unwired: 1 in]
                n288 = Multiply(x=w614, y=360.0) -> (x*y=w613:dbl)
                n289 = call-poly <vilib>:"Extract Single Tone Information.vi"("time signal in"=w623) -> ("detected phase (deg)"=w619:dbl)  [unwired: 5 in, 5 out]
                n290 = Divide(x=w613, y=w611) -> (x/y=w610:dbl)
                n291 = Subtract(x=w619, y=90.0) -> (x-y=w618:dbl)
                n292 = local read "Amplitude (V)"() -> (w604:dbl)
                n293 = local read "Frequency (Hz)"() -> (w603:dbl)
                n294 = call "angle_corrector.vi"("angle"=w618) -> ("angle corrected"=w608:dbl)  [unwired: 10 in]
                "Phase (deg)" <- w608
                n295 = for {
                  N: w611 -> [_]
                  tunnel: [w629] -> w612 mode=indexing
                  tunnel: w610 -> [w633]
                  tunnel: w608 -> [w634]
                  tunnel: w604 -> [w631]
                  tunnel: [w631] -> w607 mode=indexing
                  tunnel: w603 -> [w630]
                  tunnel: [w630] -> w605 mode=indexing
                  i -> [w635]
                  n296 = Multiply(x=w633, y=w635) -> (x*y=w632:dbl)
                  n297 = Add(x=w634, y=w632) -> (x+y=w628:dbl)
                  n298 = call "angle_corrector2.vi"("angle"=w628) -> ("angle corrected"=w629:dbl)  [unwired: 10 in]
                }
                n299 = local read "phase 2"() -> (w597:dbl)
                n300 = Replace Array Subset(array=w612, new element=w608, index=0) -> (w598:dbl[])
                n301 = Multiply(x=w597, y=-2.0) -> (x*y=w596:dbl)
                n302 = Add(x=w598, y=w596) -> (x+y=w595:dbl[])
                n303 = for {
                  tunnel: w595 -> [w627] mode=indexing
                  tunnel: [w626] -> w594 mode=indexing
                  n304 = call "angle_corrector_array.vi"("angle"=w627) -> ("angle corrected"=w626:dbl)  [unwired: 10 in]
                }
              }
            }
            n305 = Unbundle By Name(w566) -> ("Y"=w562:dbl[])
            n306 = Unbundle By Name(w565) -> ("Y"=w563:dbl[])
            n307 = Unbundle By Name(w560) -> ("Y"=w558:dbl[])
            n308 = Unbundle By Name(w559) -> ("Y"=w561:dbl[])
            n309 = case shown="True" "Boolean" {
              tunnel: w573 -> [_ w586]
              tunnel: w572 -> [_ w585]
              tunnel: w558 -> [_ w584]
              tunnel: w561 -> [_ w583]
              frame False {
              }
              frame True {
                w582 = 0 ("start index (0)")
                # "First cycle visualization"
                n310 = Divide(x=w586, y=w585) -> (x/y=w589:dbl)
                n311 = To Long Integer(number=w589) -> (32bit integer=w587:i32)
                n312 = Search 1D Array(1D array=w583, element=2.95, start index (0)=w582) -> ()  [unwired: 1 out]
                n313 = Array Subset(array=w584, index=w582, length=w587) -> (→"Cycle visualization":dbl[])
              }
            }
            n314 = Build Array(w561, w558, w562, w563) -> (w571:dbl[][])
            n315 = for {
              tunnel: w555 -> [w578] mode=indexing
              shift-right: [w578] -> _
              shift-left: _ -> [w581]
              tunnel: [w577] -> w554 mode=indexing
              n316 = local read "Pulse frequency"() -> (w579:dbl)
              n317 = Subtract(x=w578, y=w581) -> (x-y=w580:dbl)
              n318 = Multiply(x=w580, y=w579) -> (x*y=w577:dbl)
            }
          }
          frame #3 {
            n319 = case shown="0, Default" w642 {
              tunnel: w641 -> [w647 w648]
              frame 0, Default {
                "rocof0" <- w647
              }
              frame 1 {
                "rocof1" <- w648
              }
            }
            n320 = case shown="1" w642 {
              tunnel: w643 -> [w649 w650]
              frame 0, Default {
                "freq0" <- w649
              }
              frame 1 {
                "freq1" <- w650
              }
            }
            n321 = case shown="1" w642 {
              tunnel: w644 -> [w651 w652]
              frame 0, Default {
                "magnitude0" <- w651
              }
              frame 1 {
                "magnitude1" <- w652
              }
            }
            n322 = case shown="0, Default" w642 {
              tunnel: w645 -> [w653 w654]
              frame 0, Default {
                "phases0" <- w653
              }
              frame 1 {
                "phases1" <- w654
              }
            }
          }
        }
        n323 = call-poly <vilib>:"DAQmx Write.vi"("task/channels in"=w74, "data"=w72, "error in"=w92) -> ("task out"=w90:refnum<k21>, "error out"=w91:errorcluster)  [unwired: 10 in, 1 out]
        n324 = node-c288() -> ()  [unwired: 5 in, 1 out]
      }
      n325 = call <vilib>:"DAQmx Stop Task.vi"("task/channels in"=w53, "error in"=w54) -> ("task out"=w60:refnum<k21>, "error out"=w39:errorcluster)  [unwired: 12 in]
      n326 = node-c288(w68) -> (→"Iteration Duration":i64)  [unwired: 6 out]
      n327 = call <vilib>:"DAQmx Clear Task.vi"("task in"=w60, "error in"=w39) -> ("error out"=w63:errorcluster)  [unwired: 13 in]
      n328 = call <vilib>:"Simple Error Handler.vi"("type of dialog (OK msg:1)"=w65, "error in (no error)"=w63) -> ()  [unwired: 3 in, 5 out]
    }
  }
  n329 = Build Array("Loop1", "Loop2") -> (w4:string[])
  n330 = call <vilib>:"Synchronize Timed Structure Starts.vi"("timed structure names"=w4, "synchronization group name"="grupo de sincronismo") -> ()  [unwired: 8 in, 2 out]
  n331 = case shown="True" "Serial communication" {
    selector: "Serial communication" -> [_ w670]
    tunnel: "Loop2" -> [_ w671]
    frame False {
    }
    frame True {
      n332 = case shown="True" w670 {
        tunnel: [_ w705] -> w688
        tunnel: [_ w697] -> w687
        frame False {
        }
        frame True {
          n333 = call-poly "VISA Configure Serial Port"("VISA resource name"="Porta", "timeout (10sec)"="timeout (ms)", "Enable Termination\nChar (T)"=FALSE ("Enable Termination\nChar (T)"), "baud rate (9600)"="baud rate (kB)", "data bits (8)"="data bits (8)", "parity (0:none)"="parity (0:none)", "stop bits (10: 1 bit)"="stop bits (10: 1 bit)", "flow control (0:none)"="flow control (0:none)") -> ("VISA resource name out"=w705:refnum<visa-resource-name>, "error out"=w697:errorcluster)  [unwired: 6 in]
        }
      }
      n334 = call-poly <vilib>:"DAQmx Create Timing Source.vi"("counter"=tag "Dev1/ctr0", "frequency"=1000.0) -> ("timing source out"=w673:string)  [unwired: 12 in, 1 out]
      n335 = Build Path(base path="Directory", name or relative path="File name") -> (appended path=w675:path)
      n336 = node-c288(w673, i64 0 ("Period"), 100 ("Priority"), 1 ("Processor"), w671, nitl_modes."Process missed periods, ignore original phase" ("Mode"), i64 40 ("Offset")) -> (w695:T8)  [unwired: 2 in]
      n337 = Open/Create/Replace File(file path (use dialog)=w675, operation (0:open)=T12."replace or create", access (0:read/write)=enum16{"read/write", "read-only", "write-only"}."write-only") -> (refnum out=w678:refnum<file>, error out=w679:errorcluster)  [unwired: 3 in, 1 out]
      n338 = timed-loop {
        timing: w695 -> [_]
        timing-out: [_] -> w694
        tunnel: w687 -> [w778]
        tunnel: w688 -> [w777]
        tunnel: [w776] -> w686
        tunnel: [w775] -> w685
        shift-right: [w774] -> _
        shift-left: 0 ("t") -> [w773]
        shift-right: [w736] -> _
        shift-left: 0 ("initial phase") -> [w737]
        tunnel: [w726] -> w683
        tunnel: [w725] -> w682
        tunnel: w679 -> [w724]
        tunnel: w678 -> [w723]
        i -> [w734]
        stop <- "stop" stop-if-true
        n339 = node-c288() -> (w758:errorcluster, →"Iteration Duration 2":i64)  [unwired: 1 in, 2 out]
        n340 = flat-sequence {
          tunnel: w777 -> [w819]
          tunnel: w778 -> [w820]
          tunnel: [w820] -> w754
          tunnel: [w819] -> w752
          tunnel: w773 -> [w815]
          tunnel: [w810] -> w753
          tunnel: [w834] -> w751
          tunnel: [w832] -> w750
          tunnel: [w822] -> w749
          tunnel: [w824] -> w755
          tunnel: [w840] -> w748
          tunnel: [w823] -> w756
          tunnel: [w841] -> w747
          tunnel: [w839] -> w757
          tunnel: w737 -> [w827]
          tunnel: w753 -> [w829]
          tunnel: w752 -> [w837]
          tunnel: w754 -> [w838]
          tunnel: [w825] -> w718
          tunnel: [w826] -> w713
          tunnel: w751 -> [w876]
          tunnel: w750 -> [w875]
          tunnel: w749 -> [w861]
          tunnel: w755 -> [w862]
          tunnel: w748 -> [w863]
          tunnel: w756 -> [w866]
          tunnel: w747 -> [w859]
          tunnel: w757 -> [w857]
          tunnel: [w876] -> w776
          tunnel: [w875] -> w775
          tunnel: [w865] -> w728
          tunnel: [w858] -> w729
          tunnel: [w864] -> w730
          tunnel: [w863] -> w731
          tunnel: [w860] -> w732
          tunnel: [w857] -> w733
          tunnel: [w855] -> w712
          tunnel: w718 -> [w856]
          tunnel: w713 -> [w854]
          tunnel: [w854] -> w711
          frame #0 {
            n341 = local read "Pulse frequency"() -> (w809:dbl)
            n342 = To Long Integer(number=w809) -> (32bit integer=w806:i32)
            n343 = Multiply(x=2 ("y"), y=w806) -> (x*y=w807:i32)
            n344 = Greater Or Equal?(x=w815, y=w806) -> (x >= y?=w814:bool)
            n345 = Greater Or Equal?(x=w815, y=w807) -> (x >= y?=w813:bool)
            n346 = Select(t=1, s=w814, f=0) -> (s? t:f=w811:i32)
            n347 = Wait (ms)(milliseconds to wait=u32 2) -> ()  [unwired: 1 out]
            n348 = Select(t=2, s=w813, f=w811) -> (s? t:f=w810:i32)
          }
          frame #1 {
            # "leituras"
            # "Conversor"
            n349 = VISA Flush I/O Buffer(VISA resource name=w837, error in (no error)=w838) -> (VISA resource name out=w831:refnum<visa-resource-name>, error out=w835:errorcluster)  [unwired: 1 in]
            n350 = case shown="1" w829 {
              tunnel: [w849 w850] -> w843
              frame 0, Default {
                n351 = local read "magnitude0"() -> (w849:dbl[])
              }
              frame 1 {
                n352 = local read "magnitude1"() -> (w850:dbl[])
              }
            }
            n353 = case shown="1" w829 {
              tunnel: [w851 w852] -> w844
              frame 0, Default {
                n354 = local read "phases0"() -> (w851:dbl[])
              }
              frame 1 {
                n355 = local read "phases1"() -> (w852:dbl[])
              }
            }
            n356 = case shown="0, Default" w829 {
              tunnel: [w845 w846] -> w828
              frame 0, Default {
                n357 = local read "rocof0"() -> (w845:dbl[])
              }
              frame 1 {
                n358 = local read "rocof1"() -> (w846:dbl[])
              }
            }
            n359 = case shown="0, Default" w829 {
              tunnel: [w847 w848] -> w842
              frame 0, Default {
                n360 = local read "freq0"() -> (w847:dbl[])
              }
              frame 1 {
                n361 = local read "freq1"() -> (w848:dbl[])
              }
            }
            n362 = VISA Read(VISA resource name=w831, byte count=u32 16, error in (no error)=w835) -> (VISA resource name out=w832:refnum<visa-resource-name>, read buffer=w833:string, error out=w834:errorcluster)  [unwired: 1 out]
            "read buffer" <- w833
            n363 = Index Array(array=w843, index=w827) -> (element=w841:dbl)
            n364 = Index Array(array=w828, index=w827) -> (element=w826:dbl)
            n365 = Index Array(array=w842, index=w827) -> (element=w839:dbl)
            n366 = Index Array(array=w844, index=w827) -> (element=w840:dbl)
            n367 = String To Byte Array(string=w833) -> (unsigned byte array=w830:u8[])
            n368 = call "Conversor_4dados.vi"("subarray"=w830) -> ("ROCOF"=w825:sgl, "Frequência"=w824:sgl, "Ângulo"=w823:sgl, "Módulo"=w822:sgl)  [unwired: 2 in]
            n369 = Build Array(w822, w823, w824, w825) -> (→"floating point data":sgl[])
          }
          frame #2 {
            # "correçoes"
            n370 = To Double Precision Float(number=w862) -> (double precision float=w867:dbl)
            n371 = To Double Precision Float(number=w856) -> (double precision float=w855:dbl)
            n372 = case shown="False" "RMS?" {
              tunnel: w859 -> [w877 w879]
              tunnel: [w877 w878] -> w858
              frame False {
              }
              frame True {
                n373 = Square Root(x=2.0) -> (sqrt(x)=w881:dbl)
                n374 = Divide(x=w879, y=w881) -> (x/y=w878:dbl)
              }
            }
            n375 = Add(x=w867, y="Frequency\noff-set") -> (x+y=w860:dbl)
            n376 = To Double Precision Float(number=w861) -> (double precision float=w869:dbl)
            n377 = To Double Precision Float(number=w866) -> (double precision float=w868:dbl)
            n378 = Add(x=w868, y="Angle\noff-set") -> (x+y=w864:dbl)
            n379 = Multiply(x=w869, y="Magnitude\ncoefficient") -> (x*y=w871:dbl)
            n380 = Add(x=w871, y="Magnitude\noff-set") -> (x+y=w865:dbl)
          }
        }
        n381 = local read "Pulse frequency"() -> (w764:dbl)
        n382 = Multiply(x=w764, y=u16 2) -> (x*y=w767:dbl)
        n383 = Decrement(x=w767) -> (x-1=w766:dbl)
        n384 = Equal?(x=w766, y=w773) -> (x = y?=w763:bool)
        n385 = Increment(x=w773) -> (x+1=w762:i32)
        n386 = Select(t=0, s=w763, f=w762) -> (s? t:f=w774:i32)
        n387 = local read "Pulse frequency"() -> (w760:dbl)
        n388 = Decrement(x=w760) -> (x-1=w761:dbl)
        n389 = Equal?(x=w737, y=w761) -> (x = y?=w769:bool)
        n390 = Increment(x=w737) -> (x+1=w771:i32)
        n391 = Select(t=u16 0, s=w769, f=w771) -> (s? t:f=w736:i32)
        n392 = case shown="True" "Data save" {
          tunnel: w728 -> [_ w799]
          tunnel: w730 -> [_ w798]
          tunnel: w732 -> [_ w796]
          tunnel: w733 -> [_ w795]
          tunnel: w734 -> [_ w790]
          tunnel: w731 -> [_ w797]
          tunnel: w729 -> [_ w792]
          tunnel: [_ w789] -> w727
          tunnel: w712 -> [_ w788]
          tunnel: w711 -> [_ w787]
          frame False {
          }
          frame True {
            w791 = "\t"
            n393 = feedback #12(w790) -> (w794:i32)
            n394 = feedback-in #12(w794) -> ()
            n395 = Subtract(x=w790, y=w794) -> (x-y=w793:i32)
            n396 = Format Into String(w793, w791, w799, w791, w792, w791, w798, w791, w797, w791, w796, w791, w795, w791, w788, w791, w787, "\r\n") -> (resulting string=w789:string)  [unwired: 3 in, 1 out]
          }
        }
        n397 = Initialize Array(w728, 1 ("dimension size")) -> (w715:dbl[])
        "Voltage measured" <- w715
        n398 = Initialize Array(w729, 1 ("dimension size")) -> (w716:dbl[])
        "Voltage reference" <- w716
        n399 = Initialize Array(w730, 1 ("dimension size")) -> (w706:dbl[])
        "Angle measured" <- w706
        n400 = Initialize Array(w731, 1 ("dimension size")) -> (w707:dbl[])
        "Angle reference" <- w707
        n401 = Write to Text File(file (use dialog)=w723, text=w727, error in=w724) -> (refnum out=w725:refnum<file>, error out=w726:errorcluster)  [unwired: 1 in, 1 out]
        n402 = Initialize Array(w712, 1 ("dimension size")) -> (w714:dbl[])
        "ROCOF measured" <- w714
        n403 = Initialize Array(w711, 1 ("dimension size")) -> (w719:dbl[])
        "ROCOF reference" <- w719
        n404 = Initialize Array(w732, 1 ("dimension size")) -> (w708:dbl[])
        "Frequency measured" <- w708
        n405 = Initialize Array(w733, 1 ("dimension size")) -> (w709:dbl[])
        "Frequency reference" <- w709
        n406 = case shown="True" "?" {
          tunnel: w715 -> [_ w891]
          tunnel: w716 -> [_ w890]
          frame False {
          }
          frame True {
            n407 = Build Array(w891, w890) -> (w893:dbl[][])
            n408 = Transpose 2D Array(2D array=w893) -> (transposed array=→"Magnitude measures (V)":dbl[][])
          }
        }
        n409 = case shown="True" "?" {
          tunnel: w707 -> [_ w886]
          tunnel: w706 -> [_ w887]
          frame False {
          }
          frame True {
            n410 = Build Array(w887, w886) -> (w889:dbl[][])
            n411 = Transpose 2D Array(2D array=w889) -> (transposed array=→"Phase measures (º)":dbl[][])
          }
        }
        n412 = case shown="True" "?" {
          tunnel: w714 -> [_ w783]
          tunnel: w719 -> [_ w782]
          frame False {
          }
          frame True {
            n413 = Build Array(w783, w782) -> (w784:dbl[][])
            n414 = Transpose 2D Array(2D array=w784) -> (transposed array=→"ROCOF (Hz/s)":dbl[][])
          }
        }
        n415 = case shown="True" "?" {
          tunnel: w709 -> [_ w884]
          tunnel: w708 -> [_ w883]
          frame False {
          }
          frame True {
            n416 = Build Array(w883, w884) -> (w885:dbl[][])
            n417 = Transpose 2D Array(2D array=w885) -> (transposed array=→"Frequency measures (Hz)":dbl[][])
          }
        }
        n418 = case shown="True" "Boolean 3" {
          tunnel: w716 -> [_ w801]
          tunnel: w715 -> [_ w803]
          tunnel: w706 -> [_ w802]
          tunnel: w707 -> [_ w800]
          frame False {
          }
          frame True {
            n419 = call-poly <vilib>:"Plot Helper.vi"("radius vector"=w803, "theta vector"=w802) -> ("2D Plot Class Obj Array out"=w804:refnum<class "2D Plot Datatype.lvclass">[])  [unwired: 2 in, 7 out]
            n420 = call-poly <vilib>:"Plot Helper.vi"("radius vector"=w801, "theta vector"=w800, "2D Plot Class Obj Array in"=w804) -> ("2D Plot Class Obj Array out"=→"Phasors visualization":refnum<class "2D Plot Datatype.lvclass">[])  [unwired: 1 in, 7 out]
          }
        }
        n421 = case shown="True" "?" {
          tunnel: w707 -> [_ w781]
          tunnel: w706 -> [_ w780]
          frame False {
          }
          frame True {
            n422 = Subtract(x=w781, y=w780) -> (x-y=→"Phase measures (º) 2":dbl[])
          }
        }
        n423 = node-c288(w758) -> ()  [unwired: 1 out]
      }
      n424 = node-c288(w694) -> ()  [unwired: 1 out]
      n425 = Close File(refnum=w682, error in=w683) -> ()  [unwired: 2 out]
      n426 = VISA Close(VISA resource name=w685, error in (no error)=w686) -> ()  [unwired: 1 out]
    }
  }
  n427 = case shown="True" TRUE {
    frame False {
    }
    frame True {
      n428 = while {
        stop <- FALSE stop-if-true
        n429 = case shown="\"Real-Time Data\"" "Tab Control" {
          frame "Communication", Default {
          }
          frame "Real-Time Data" {
            n430 = local read "Pulse frequency"() -> (w914:dbl)
            n431 = Initialize Array(0.0 ("element"), w914) -> (w913:dbl[])
            "initialized array" <- w913
            n432 = while {
              shift-right: [w953] -> _
              shift-left: 0 -> [w930]
              tunnel: w914 -> [w952]
              tunnel: w913 -> [w927]
              stop <- w943 stop-if-true
              # "Escrevem nos controles da  aba principal"
              # "Controles da aba Real-Time Data"
              # "Indicadores da aba Real-Time Data"
              n433 = local read "Phase (deg)"() -> (→"Phase (degrees) 2":dbl)
              n434 = Wait (ms)(milliseconds to wait=u32 30) -> ()  [unwired: 1 out]
              n435 = local read "ROCOF measured"() -> (w928:dbl[])
              n436 = local read "ROCOF reference"() -> (w929:dbl[])
              n437 = local read "Frequency reference"() -> (w936:dbl[])
              n438 = local read "Voltage measured"() -> (w924:dbl[])
              n439 = local read "Frequency measured"() -> (w935:dbl[])
              n440 = local read "Angle measured"() -> (w933:dbl[])
              n441 = local read "Angle reference"() -> (w934:dbl[])
              n442 = local read "Voltage reference"() -> (w923:dbl[])
              n443 = Equal?(x=w952, y=w930) -> (x = y?=w944:bool)
              n444 = Increment(x=w930) -> (x+1=w955:i32)
              n445 = feedback #13(w927) -> (w961:dbl[])
              n446 = Replace Array Subset(array=w961, new element=w923, index=w930) -> (w947:dbl[])
              n447 = feedback-in #13(w947) -> ()
              n448 = feedback #14(w927) -> (w960:dbl[])
              n449 = Replace Array Subset(array=w960, new element=w924, index=w930) -> (w948:dbl[])
              n450 = feedback-in #14(w948) -> ()
              n451 = feedback #15(w927) -> (w957:dbl[])
              n452 = Replace Array Subset(array=w957, new element=w935, index=w930) -> (w945:dbl[])
              n453 = feedback-in #15(w945) -> ()
              n454 = feedback #16(w927) -> (w956:dbl[])
              n455 = Replace Array Subset(array=w956, new element=w936, index=w930) -> (w946:dbl[])
              n456 = feedback-in #16(w946) -> ()
              n457 = feedback #17(w927) -> (w959:dbl[])
              n458 = Replace Array Subset(array=w959, new element=w933, index=w930) -> (w949:dbl[])
              n459 = feedback-in #17(w949) -> ()
              n460 = feedback #18(w927) -> (w958:dbl[])
              n461 = Replace Array Subset(array=w958, new element=w934, index=w930) -> (w950:dbl[])
              n462 = feedback-in #18(w950) -> ()
              n463 = feedback #19(w927) -> (w932:dbl[])
              n464 = Replace Array Subset(array=w932, new element=w928, index=w930) -> (w926:dbl[])
              n465 = feedback-in #19(w926) -> ()
              n466 = feedback #20(w927) -> (w931:dbl[])
              n467 = Replace Array Subset(array=w931, new element=w929, index=w930) -> (w925:dbl[])
              n468 = feedback-in #20(w925) -> ()
              n469 = Select(t=0, s=w944, f=w955) -> (s? t:f=w953:i32)
              n470 = case shown="True" w944 {
                selector: w944 -> [_ w973]
                tunnel: w950 -> [_ w989]
                tunnel: w949 -> [_ w988]
                tunnel: w948 -> [_ w963]
                tunnel: w947 -> [_ w972]
                tunnel: w946 -> [_ w983]
                tunnel: w945 -> [_ w982]
                tunnel: [FALSE w973] -> w943
                tunnel: w926 -> [_ w968]
                tunnel: w925 -> [_ w967]
                frame False {
                }
                frame True {
                  n471 = call "Statistical measure - basics - 4.vi"("Data measured"=w968, "Data reference"=w967) -> ("Statistcs"=w966:T13)  [unwired: 12 in, 1 out]
                  n472 = Add Array Elements(numeric array=w963) -> (sum=w971:dbl)
                  n473 = Array Size(array=w963) -> (size(s)=w970:i32)
                  n474 = call "Statistical measure - basics percentual - 1.vi"("Data measured"=w972, "Data reference"=w963) -> ("Statistcs"=w984:T13)  [unwired: 12 in, 1 out]
                  n475 = call "Statistical measure - basics - 1.vi"("Data measured"=w988, "Data reference"=w989) -> ("Statistcs"=w991:T13)  [unwired: 12 in, 1 out]
                  n476 = call "Statistical measure - basics - 3.vi"("Data measured"=w982, "Data reference"=w983) -> ("Statistcs"=w981:T13)  [unwired: 12 in, 1 out]
                  n477 = call "TVE.vi"("Angle reference"=w989, "Angle measured"=w988, "Voltage reference"=w963, "Voltage measured"=w972) -> ("Array"=w986:dbl[])
                  n478 = local read "initialized array"() -> (w987:dbl[])
                  n479 = Unbundle By Name(w966) -> ("max dev"=→"max rocof":dbl, "mean dev"=→"mean rocof":dbl)
                  n480 = Unbundle By Name(w984) -> ("max dev"=→"max magnitude":dbl, "mean dev"=→"mean dev":dbl)
                  n481 = Divide(x=w971, y=w970) -> (x/y=→"Media":dbl)
                  n482 = Unbundle By Name(w991) -> ("max dev"=→"max phase":dbl, "mean dev"=→"mean phase":dbl)
                  n483 = Unbundle By Name(w981) -> ("max dev"=→"max freq":dbl, "mean dev"=→"mean freq":dbl)
                  n484 = call "Statistical measure - basics - 2.vi"("Data measured"=w986, "Data reference"=w987) -> ("Statistcs"=w985:T13)  [unwired: 12 in, 1 out]
                  n485 = Unbundle By Name(w985) -> ("max dev"=→"max tve":dbl, "mean dev"=→"mean tve":dbl)
                }
              }
              n486 = local write "Amplitude (%)"("Amp. (%) 2") -> ()
              n487 = local write "Interf.\nFrequency (Hz)"("Interf. Frequency 2") -> ()
              n488 = local write "Interf.\nAmplitude (%)"("amplitude") -> ()
              n489 = local write "Interference"("Interference 2") -> ()
              n490 = local write "Order"("Order 2") -> ()
              n491 = local write "Harmonics"("Harmonics 2") -> ()
              n492 = local write "Offset"("Offset 2") -> ()
              n493 = local write "Phase"("Phase 2") -> ()
              n494 = local write "Amplitude"("Amplitude 2") -> ()
              n495 = local write "Frequency"("Frequency 2") -> ()
              n496 = local write "reset\nphase?"("reset signal 2") -> ()
            }
          }
          frame "Measure statistics" {
          }
        }
        n497 = Wait (ms)(milliseconds to wait=u32 1000) -> ()  [unwired: 1 out]
      }
    }
  }
